vi "STM Command Based Example - Server.vi"() -> ()   [LabVIEW 2010]
doc: "This example demonstrates how to use STM with TCP to implement a command based communications application. \n\nThe server receives messages from the client on the type of signals to generate (frequency, FFT window type) and then sends time domain and spectral data to the client.\n\nThe server must be started first."
uses:
  vi.lib/NI/STM/SubVIs/MetaDataElement.ctl
  vi.lib/NI/STM/TCP/TCP Read Options.ctl
  vi.lib/NI/STM/TCP/Write Meta Data (TCP Ref).vi
  vi.lib/NI/STM/TCP/Get Connection Reference (TCP).vi
  vi.lib/NI/STM/TCP/Write Meta Data (TCP Clst).vi
  <vilib>/measure/maspectr.llb/FFT Power Spectrum for 1 Chan.vi
  vi.lib/NI/STM/TCP/Write Message (TCP).vi
  vi.lib/NI/STM/TCP/Read Message (TCP).vi
  <vilib>/measure/NI_MAPro.lvlib
  <vilib>/measure/NI_MABase.lvlib
  vi.lib/NI/STM/NI STM.lvlib
panel:
  out "Window":T1(ring)
  out "error  out":errorcluster
  in  "stop":bool
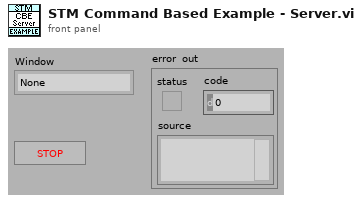
[diagram p1: front panel]
types:
  T1 = enum16{"None ", "Hanning", "Hamming", "Blackman-Harris", "Exact Blackman", "Blackman", "Flat Top", "4 Term B-Harris ", "7 Term B-Harris", "Low Sidelobe"}
  T2 = typedef "NI STM.lvlib/MetaDataElement.ctl" = string
  T3 = typedef "NI STM.lvlib/TCP Connection Info.ctl" = cluster{"connection ID":refnum<k5>, "meta data":T2[]}
  T4 = typedef "Command Based Example Queue Refs.ctl" = cluster{"Data Queue":refnum<queue>, "Frequency Queue":refnum<queue>}
  T5 = typedef "NI STM.lvlib/TCP Read Options.ctl" = cluster{"ignore timeout error":bool, "timeout ms (1000)":i32}
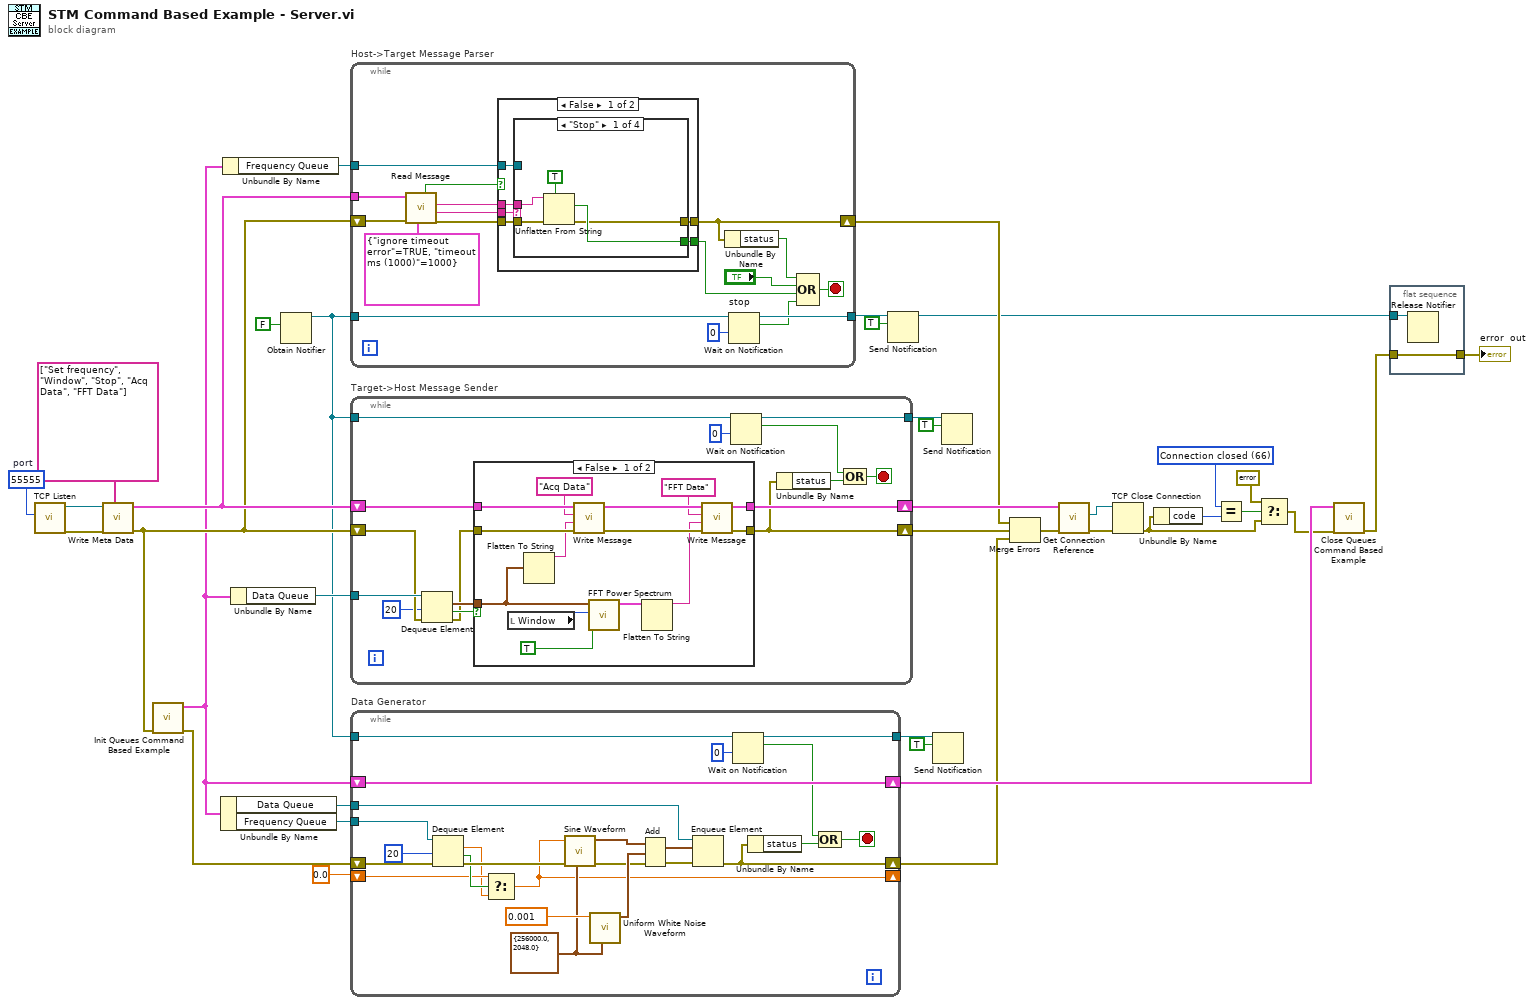
[diagram p0: block diagram]
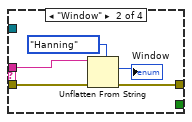
[diagram p3: hidden frame]
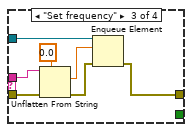
[diagram p4: hidden frame]
diagram:
  w4 = 66 items=["No Error", "Argument Error", "Memory Full", "Out of Zone", "End of File", "File Already Open", "Generic File IO Error", "File Not Found", "File Permission Error", "Disk Full", "Duplicate Path", "Too Many Files Open", "Not Enabled", "Resource File Not Found", "Cannot Add Resource", "Resource Not Found", "Image Not Found", "Image Memory Error", "Pen Does Not Exist", "Config Bad Type", "Config Token Not Found", "Config Parse Error", "Config Memory Error", "Bad External Code Format", "Bad External Code Offset", "External Code Not Present", "Null Window", "Destroy Window Mixup", "Null Menu", "Print Aborted", "Bad Print Record", "Print Driver Error", "Windows Error During Print", "Memory Error During Print", "Print Dialog Error", "Generic Print Error", "Invalid Device Refnum", "Device Not Found", "Device Parameter Error", "Device Unit Error", "Can't Open Device", "Device Call Aborted", "Generic Error", "Cancelled By User", "Object ID Too Low", "Object ID Too High", "Object Not In Heap", "Unknown Heap", "Bad DefProc ID", "DefProc Not In Table", "Message Out Of Range", "Null Method", "Unknown Message", "Manager Call Not Supported", "Bad address", "Connection In progress", "Connection timed out", "Connection is already in progress", "Network attribute not supported", "Network error", "Address in use", "System out of memory", "Connection aborted", "Connection refused", "Connection is not connected", "Connection is already connected", "Connection closed", "Initialize error (interapplication manager)", "Bad occurrence", "Wait on unbound occurrence handler", "Occurrence queue overflow", "Bad path", "Semaphore not signaled", "Unrecognized type (interapplication manager)"] ("1st Error to Convert")
  w38 = u16 55555  # port
  n1 = call <vilib>:"TCP Listen.vi"("port"=w38) -> ("error out"=w36:errorcluster, "connection ID"=w37:refnum<k5>)  [unwired: 3 in, 6 out]
  n2 = call-poly "Write Meta Data.vi"("meta data"=T2[] ["Set frequency", "Window", "Stop", "Acq Data", "FFT Data"] ("Meta data"), "error in"=w36, "connection ID"=w37) -> ("error out"=w34:errorcluster, "connection info out"=w35:T3)  [unwired: 2 in, 5 out]
  n3 = call "Init Queues Command Based Example.vi"("error in (no error)"=w34) -> ("error out"=w28:errorcluster, "Queue Refs"=w27:T4)  [unwired: 9 out]
  n4 = Unbundle By Name(w27) -> ("Data Queue"=w31:refnum<queue>, "Frequency Queue"=w30:refnum<queue>)
  n5 = Unbundle By Name(w27) -> ("Frequency Queue"=w32:refnum<queue>)
  n6 = Unbundle By Name(w27) -> ("Data Queue"=w33:refnum<queue>)
  n7 = Obtain Notifier(notification data type=FALSE) -> (notifier out=w12:refnum<notifier>)  [unwired: 3 in, 2 out]
  n8 = while "Host->Target Message Parser" {
    tunnel: w35 -> [w55]
    tunnel: w32 -> [w50]
    shift-right: [w45] -> w20
    shift-left: w34 -> [w54]
    tunnel: w12 -> [w47]
    tunnel: [w41] -> w16
    stop <- w42 stop-if-true
    n9 = call-poly "Read Message.vi"("options"=T5 {"ignore timeout error"=TRUE, "timeout ms (1000)"=1000} ("Options"), "error in"=w54, "connection info in"=w55) -> ("error out"=w49:errorcluster, "name"=w53:T2, "data string"=w52:string, "timed out?"=w51:bool)  [unwired: 2 in, 3 out]
    n10 = case shown="False" w51 {
      tunnel: w53 -> [w57 _]
      tunnel: w52 -> [w61 _]
      tunnel: w50 -> [w60 _]
      tunnel: w49 -> [w59 w80]
      tunnel: [w58 w80] -> w45
      tunnel: [w56 _] -> w39
      frame False {
        n11 = case shown="\"Stop\"" w57 {
          tunnel: w61 -> [w65 w69 w75 _]
          tunnel: w60 -> [_ _ w78 _]
          tunnel: w59 -> [w64 w68 w74 w79]
          tunnel: [w62 w67 w72 w79] -> w58
          tunnel: [w63 _ _ _] -> w56
          frame "Stop" {
            n12 = Unflatten From String(type=TRUE, binary string=w65, error in (no error)=w64) -> (value=w63:bool, error out=w62:errorcluster)  [unwired: 1 in, 2 out]
          }
          frame "Window" {
            n13 = Unflatten From String(type=T1."Hanning" ("window"), binary string=w69, error in (no error)=w68) -> (value=→"Window":T1, error out=w67:errorcluster)  [unwired: 1 in, 2 out]
          }
          frame "Set frequency" {
            n14 = Unflatten From String(type=0.0, binary string=w75, error in (no error)=w74) -> (value=w76:dbl, error out=w73:errorcluster)  [unwired: 1 in, 2 out]
            n15 = Enqueue Element(queue=w78, element=w76, error in (no error)=w73) -> (error out=w72:errorcluster)  [unwired: 3 out]
          }
          frame Default {
          }
        }
      }
      frame True {
      }
    }
    n16 = Unbundle By Name(w45) -> ("status"=w44:bool)
    n17 = Wait on Notification(notifier=w47, timeout in ms (-1)=0) -> (notifier out=w41:refnum<notifier>, notification=w40:bool)  [unwired: 2 in, 2 out]
    n18 = Compound Arithmetic op=OR(w44, "stop", w39, w40) -> (w42:bool)
  }
  n19 = while "Target->Host Message Sender" {
    tunnel: w33 -> [w93]
    shift-right: [w85] -> w22
    shift-left: w34 -> [w90]
    shift-right: [w94] -> w25
    shift-left: w35 -> [w95]
    tunnel: w12 -> [w86]
    tunnel: [w81] -> w13
    stop <- w82 stop-if-true
    n20 = Dequeue Element(queue=w93, timeout in ms (-1)=20, error in (no error)=w90) -> (element=w92:waveform(dbl), timed out?=w91:bool, error out=w89:errorcluster)  [unwired: 1 out]
    n21 = case shown="False" w91 {
      tunnel: w95 -> [w109 w111]
      tunnel: w89 -> [w108 w110]
      tunnel: [w104 w111] -> w94
      tunnel: [w106 w110] -> w85
      tunnel: w92 -> [w96 _]
      frame False {
        n22 = local read "Window"() -> (w98:T1)
        n23 = Flatten To String(anything=w96) -> (data string=w101:string)  [unwired: 1 in, 4 out]
        n24 = call-poly "Write Message.vi"("error in"=w108, "data"=w101, "name"="Acq Data" ("Name"), "connection info in"=w109) -> ("error out"=w103:errorcluster, "connection info out"=w105:T3)  [unwired: 1 in, 5 out]
        n25 = call-poly <vilib>:"FFT Power Spectrum.vi"("dB On (F)"=TRUE, "window"=w98, "time signal"=w96) -> ("power spectrum"=w100:cluster{"f0":dbl, "df":dbl, "magnitude":dbl[]})  [unwired: 3 in, 5 out]
        n26 = Flatten To String(anything=w100) -> (data string=w99:string)  [unwired: 1 in, 4 out]
        n27 = call-poly "Write Message.vi"("error in"=w103, "data"=w99, "name"="FFT Data" ("Name"), "connection info in"=w105) -> ("error out"=w106:errorcluster, "connection info out"=w104:T3)  [unwired: 1 in, 5 out]
      }
      frame True {
      }
    }
    n28 = Wait on Notification(notifier=w86, timeout in ms (-1)=0) -> (notifier out=w81:refnum<notifier>, notification=w83:bool)  [unwired: 2 in, 2 out]
    n29 = Unbundle By Name(w85) -> ("status"=w84:bool)
    n30 = Compound Arithmetic op=OR(w83, w84) -> (w82:bool)
  }
  n31 = while "Data Generator" {
    tunnel: w31 -> [w135]
    tunnel: w30 -> [w134]
    shift-right: [w119] -> _
    shift-left: 0.0 -> [w121]
    shift-right: [w116] -> w21
    shift-left: w28 -> [w133]
    shift-right: [w126] -> w26
    shift-left: w27 -> [w126]
    tunnel: w12 -> [w117]
    tunnel: [w112] -> w10
    stop <- w113 stop-if-true
    w127 = cluster{"Fs":dbl, "#s":dbl} {"Fs"=256000.0, "#s"=2048.0} ("sampling info")
    n32 = Dequeue Element(queue=w134, timeout in ms (-1)=20, error in (no error)=w133) -> (element=w120:dbl, timed out?=w122:bool, error out=w132:errorcluster)  [unwired: 1 out]
    n33 = Select(t=w121, s=w122, f=w120) -> (s? t:f=w119:dbl)
    n34 = call <vilib>:"Sine Waveform.vi"("sampling info"=w127, "error in (no error)"=w132, "frequency"=w119) -> ("error out"=w125:errorcluster, "signal out"=w130:waveform(dbl))  [unwired: 4 in, 3 out]
    n35 = call <vilib>:"Uniform White Noise Waveform.vi"("sampling info"=w127, "amplitude"=0.001 ("Amplitude")) -> ("signal out"=w129:waveform(dbl))  [unwired: 3 in, 6 out]
    n36 = Add(1:w129, 2:w130, 4:w125) -> (0:w128:waveform(dbl), 3:w124:errorcluster)
    n37 = Enqueue Element(queue=w135, element=w128, error in (no error)=w124) -> (error out=w116:errorcluster)  [unwired: 3 out]
    n38 = Wait on Notification(notifier=w117, timeout in ms (-1)=0) -> (notifier out=w112:refnum<notifier>, notification=w114:bool)  [unwired: 2 in, 2 out]
    n39 = Unbundle By Name(w116) -> ("status"=w115:bool)
    n40 = Compound Arithmetic op=OR(w114, w115) -> (w113:bool)
  }
  n41 = Send Notification(notification=TRUE, notifier=w16) -> (notifier out=w9:refnum<notifier>)  [unwired: 1 in, 1 out]
  n42 = Send Notification(notification=TRUE, notifier=w10) -> ()  [unwired: 1 in, 2 out]
  n43 = Send Notification(notification=TRUE, notifier=w13) -> ()  [unwired: 1 in, 2 out]
  n44 = Merge Errors(w20, w22, w21) -> (w19:errorcluster)
  n45 = call-poly "Get Connection Reference.vi"("error in"=w19, "connection info in"=w25) -> ("error out"=w23:errorcluster, "connection ID out"=w24:refnum<k5>)  [unwired: 8 out]
  n46 = TCP Close Connection(connection ID=w24, error in (no error)=w23) -> (error out=w3:errorcluster)  [unwired: 2 out]
  n47 = Unbundle By Name(w3) -> ("code"=w6:i32)
  n48 = Equal?(x=w4, y=w6) -> (x = y?=w5:bool)
  n49 = Select(t=errorcluster {"status"=FALSE, "code"=0, "source"=""}, s=w5, f=w3) -> (s? t:f=w2:errorcluster)
  n50 = call "Close Queues Command Based Example.vi"("error in (no error)"=w2, "FIFOs In"=w26) -> ("error out"=w8:errorcluster)  [unwired: 9 out]
  n51 = flat-sequence {
    tunnel: w9 -> [w137]
    tunnel: w8 -> [w136]
    tunnel: [w136] -> w7
    frame #0 {
      n52 = Release Notifier(notifier=w137) -> ()  [unwired: 2 in, 3 out]
    }
  }
  "error  out" <- w7
